vi "Stop Core.vi"(10 "final error code":i32 caption="最终错误代码", 11 "ErrorHanlder in":refnum<class "ErrorHanlder.lvclass"> caption="操作者输入") -> (3 "ErrorHanlder out":refnum<class "ErrorHanlder.lvclass"> caption="操作者输出")   [LabVIEW 2019, in "ErrorHanlder.lvlib" / "ErrorHanlder.lvclass"]
doc: "(<B>文件名</B>: Actor Framework.lvlib:Actor.lvclass:Stop Core.vi)\n\n定义停止前操作者的动作。Use the <B>final error code</B> input to determine whether the actor shut down in response to an error.\n\nBy default, this method passes the Stop message along to all auto-stop nested actors.A descendant class may override this method to define additional behavior, such as shutting down any processes the actor initiated in its override of the Actor Core method."
uses:
  ErrorHanlder.lvclass
  <vilib>/ActorFramework/Actor/Actor.lvclass
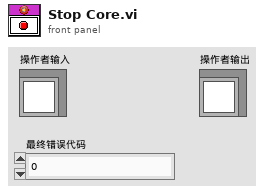
[diagram p1: front panel]
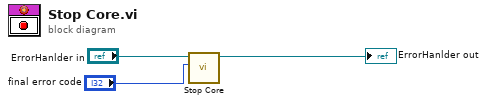
[diagram p0: block diagram]
diagram:
  n1 = call-parent "Stop Core.vi"("final error code"="final error code", "Actor in"="ErrorHanlder in") -> ("Actor out"=→"ErrorHanlder out":refnum<class "ErrorHanlder.lvclass">)  [unwired: 9 in]
